vi "20170323 - FPGA backup.vi"() -> ()   [LabVIEW 2016]
uses:
  <vilib>/rvi/Emulation/niFpgaGetClockAttributes.vi
  <vilib>/rvi/Emulation/niFpgaSctlEmulationGetInTimedLoop.vi
  <vilib>/rvi/Emulation/niFpgaEmulationReportErrorSimple.vi
  <vilib>/rvi/eio/common/nirviEmuTemplateMethod_errors.vi
  <vilib>/rvi/Emulation/niFpgaCriticalErrorInLSC.vi
  <vilib>/rvi/interface/RandomDataEmulation/niFpgaRandomDataHandleErrors.vi
  <vilib>/eio/EIONode/EIONode.xnode
  <vilib>/rvi/DataTransferAndStorage/Container/XNode/niFpgaContainer.xnode
  <vilib>/rvi/interface/RandomDataEmulation/nirviRandomDataFpgaReadWriteTemplate.vi
panel:
  in  "DOIFIFO Loop Period (us)":u32 caption="Count(uSec)"
  in  "AO1 Loop Period (us)":u32
  in  "Connector0/DIO0":bool
  in  "DIO Loop Period (us)":u32 caption="Count(uSec)"
  in  "freq":u32
  in  "AO Loop Period (us)":u32=1
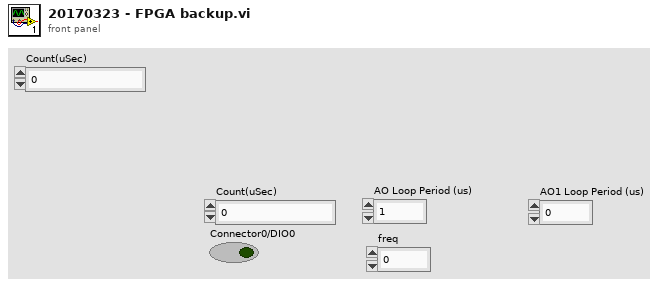
[diagram p1: front panel]
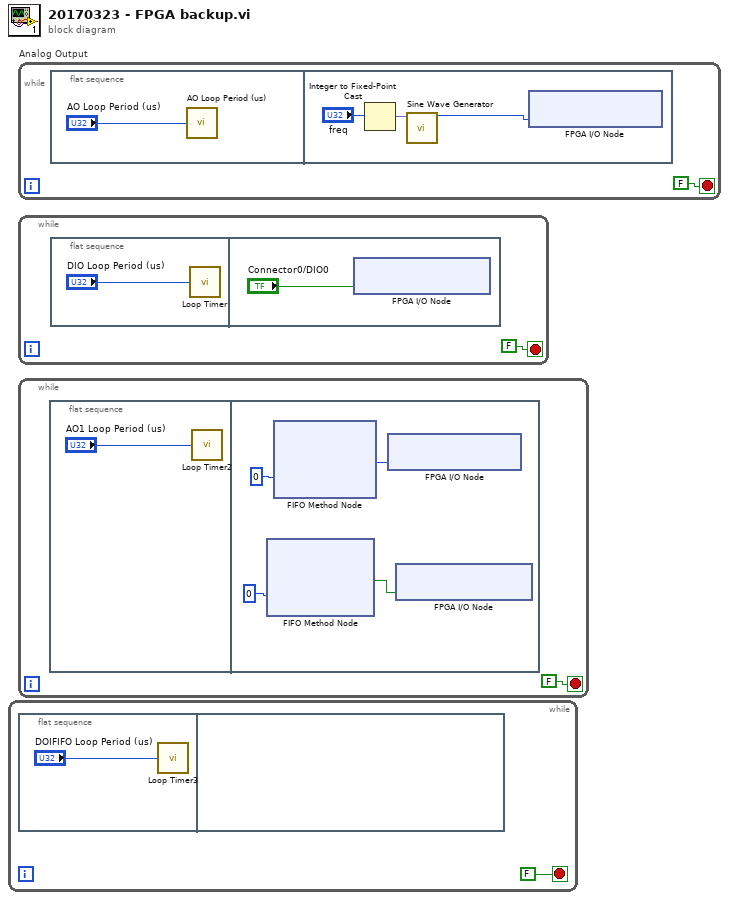
[diagram p0: block diagram]
diagram:
  n1 = while {
    stop <- FALSE stop-if-true
    n2 = flat-sequence {
      frame #0 {
        n3 = call "Loop Timer3"("Count(uSec)"="DOIFIFO Loop Period (us)") -> ()  [unwired: 1 out]
      }
      frame #1 {
      }
    }
  }
  n4 = while "Analog Output" {
    stop <- FALSE stop-if-true
    n5 = flat-sequence {
      frame #0 {
        n6 = call "AO Loop Period (us)"("Count(uSec)"="AO Loop Period (us)") -> ()  [unwired: 1 out]
      }
      frame #1 {
        n7 = Integer to Fixed-Point Cast(integer="freq") -> (fixed-point=w6:fxp<+,32,0>)  [unwired: 1 in]
        n8 = call "Sine Wave Generator"("frequency (periods/tick)"=w6) -> ("sine out"=w7:i16)  [unwired: 14 in]
        n9 = xnode "FPGA I/O Node"("Connector0/AO0"=w7) -> ()  [unwired: 1 in, 1 out]
      }
    }
  }
  n10 = while {
    stop <- FALSE stop-if-true
    n11 = flat-sequence {
      frame #0 {
        n12 = call "Loop Timer"("Count(uSec)"="DIO Loop Period (us)") -> ()  [unwired: 1 out]
      }
      frame #1 {
        n13 = xnode "FPGA I/O Node"("Connector0/DIO0"="Connector0/DIO0") -> ()  [unwired: 1 in, 1 out]
      }
    }
  }
  n14 = while {
    stop <- FALSE stop-if-true
    n15 = flat-sequence {
      frame #0 {
        n16 = call "Loop Timer2"("Count(uSec)"="AO1 Loop Period (us)") -> ()  [unwired: 1 out]
      }
      frame #1 {
        n17 = xnode ("FIFO Method Node")("Timeout"=0) -> ("Element"=w14:bool)  [unwired: 1 in, 2 out]
        n18 = xnode ("FIFO Method Node")("Timeout"=0) -> ("Element"=w16:i16)  [unwired: 1 in, 2 out]
        n19 = xnode "FPGA I/O Node"("Connector0/AO1"=w16) -> ()  [unwired: 1 in, 1 out]
        n20 = xnode "FPGA I/O Node"("Connector0/DIO1"=w14) -> ()  [unwired: 1 in, 1 out]
      }
    }
  }
